vi "一维数组操作函数.vi"() -> ()   [LabVIEW 2010]
panel:
  out "抽取数组3":i32[](array[numeric])
  out "抽取数组2":i32[](array[numeric])
  out "抽取数组1":i32[](array[numeric])
  out "交织后的数组":i32[](array[numeric])
  out "分数索引":dbl format="%.2f"
  out "插值结果":dbl format="%.2f"
  out "排序后的数组":i32[](array[numeric])
  out "拆分的子数组2":i32[](array[numeric])
  out "拆分的子数组1":i32[](array[numeric])
  out "搜索到的位置":i32
  out "反转后的数组":i32[](array[numeric])
  out "移位后的数组":i32[](array[numeric])
  out "移位后的数组":i32[](array[numeric])
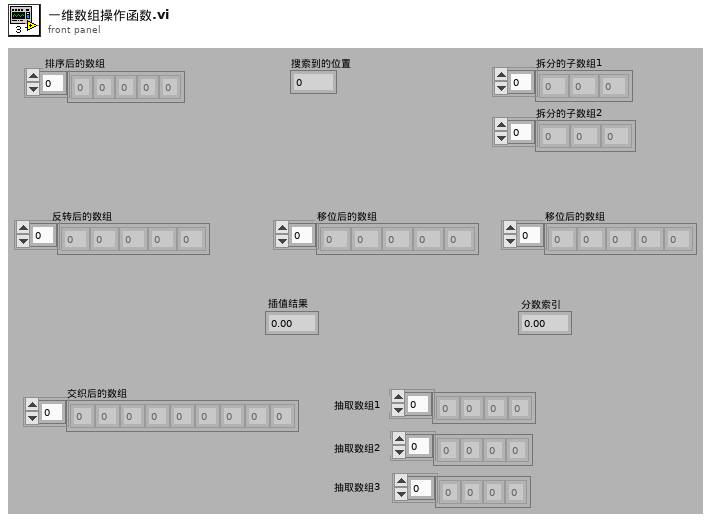
[diagram p1: front panel]
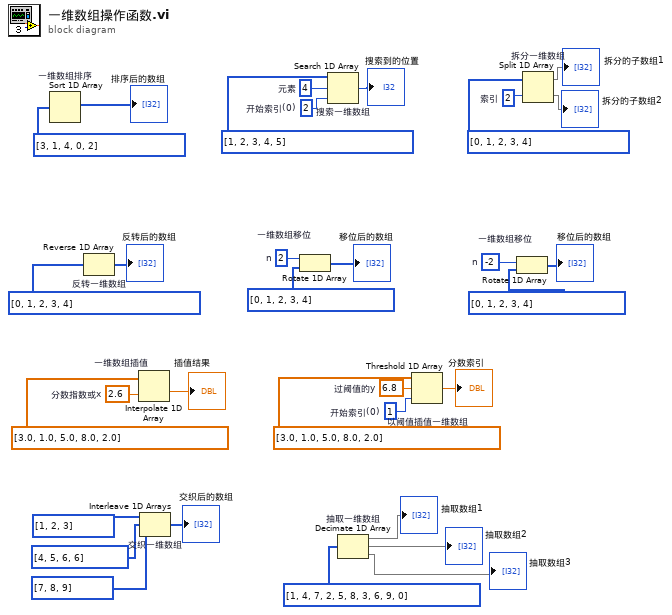
[diagram p0: block diagram]
diagram:
  w1 = 1  # 开始索引(0)
  w2 = 6.8  # 过阈值的y
  w3 = 2  # n
  w4 = 2.6  # 分数指数或x
  w5 = -2  # n
  w6 = 2  # 索引
  w7 = 2  # 开始索引(0)
  w26 = 4  # 元素
  n1 = Sort 1D Array "一维数组排序"(array=i32[] [3, 1, 4, 0, 2] ("子数组")) -> (sorted array=→"排序后的数组":i32[])
  n2 = Reverse 1D Array "反转一维数组"(array=i32[] [0, 1, 2, 3, 4] ("子数组")) -> (reversed array=→"反转后的数组":i32[])
  n3 = Interpolate 1D Array "一维数组插值"(1:w4, 2:dbl[] [3.0, 1.0, 5.0, 8.0, 2.0] ("子数组")) -> (0:→"插值结果":dbl)
  n4 = Interleave 1D Arrays "交织一维数组"(i32[] [1, 2, 3], i32[] [4, 5, 6, 6], i32[] [7, 8, 9]) -> (→"交织后的数组":i32[])
  n5 = Rotate 1D Array "一维数组移位"(1:i32[] [0, 1, 2, 3, 4] ("子数组"), 2:w3) -> (0:→"移位后的数组":i32[])
  n6 = Search 1D Array "搜索一维数组"(1D array=i32[] [1, 2, 3, 4, 5] ("子数组"), element=w26, start index (0)=w7) -> (index of element=→"搜索到的位置":i32)
  n7 = Decimate 1D Array "抽取一维数组"(i32[] [1, 4, 7, 2, 5, 8, 3, 6, 9, 0] ("插接后的数组")) -> (→"抽取数组1":i32[], →"抽取数组2":i32[], →"抽取数组3":i32[])
  n8 = Threshold 1D Array "以阈值插值一维数组"(1:w1, 2:w2, 3:dbl[] [3.0, 1.0, 5.0, 8.0, 2.0] ("子数组")) -> (0:→"分数索引":dbl)
  n9 = Rotate 1D Array "一维数组移位"(1:i32[] [0, 1, 2, 3, 4] ("子数组"), 2:w5) -> (0:→"移位后的数组":i32[])
  n10 = Split 1D Array "拆分一维数组"(array=i32[] [0, 1, 2, 3, 4] ("子数组"), index=w6) -> (first subarray=→"拆分的子数组1":i32[], second subarray=→"拆分的子数组2":i32[])
